vi "Save Config File.vi"(8 "error in (no error)":errorcluster, 10 "file path":path, 11 "DSF Configuration Reference in":T1) -> (0 "error out":errorcluster, 2 "file path out":path, 3 "DSF Configuration Reference out":T1)   [LabVIEW 2017, in "DSF Core.lvlib" / "Configuration Session.lvclass"]
uses:
  Configuration Session.lvclass
  Internal DSF Channel with ID.ctl
  Internal DSF Transfer with ID.ctl
  Typedefs/DSF Timing Info.ctl
  DSF Core.lvlib
  Internal DSF Group with ID.ctl
  Internal DSF Plugin with ID.ctl
  Typedefs/DSF Version Info.ctl
  Internal DSF Settings with ID.ctl
  Internal DSF Configuration.ctl
  Internal DSF Channel Info.ctl
  Internal DSF Transfer Info.ctl
  Internal DSF Group Info.ctl
  Internal DSF Plugin Info.ctl
  Internal DSF Settings Info.ctl
  DSF Config Data.ctl
  DSF Config Data Ref.ctl
  Typedefs/DSF Settings Info.ctl
  Typedefs/DSF Engine Plugin Thread Configuration.ctl
  Typedefs/DSF Engine Framework Configuration.ctl
  Typedefs/DSF Direction.ctl
  Typedefs/DSF Byte Order.ctl
  Typedefs/DSF Data Type.ctl
  Typedefs/DSF Engine Channel Configuration.ctl
  Typedefs/DSF Engine Transfer Configuration.ctl
  Typedefs/DSF Timeout Behavior.ctl
  Typedefs/DSF Engine Transfer Group Configuration.ctl
  Typedefs/DSF Engine Plugin Configuration.ctl
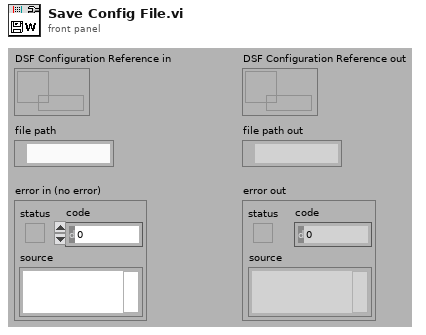
[diagram p1: front panel]
types:
  T1 = typedef "DSF Core.lvlib/Configuration Session.lvclass/DSF Config Data Ref.ctl" = refnum<data-value>
  T2 = enum16{"open", "replace", "create", "open or create", "replace or create", "replace or create with confirmation"}
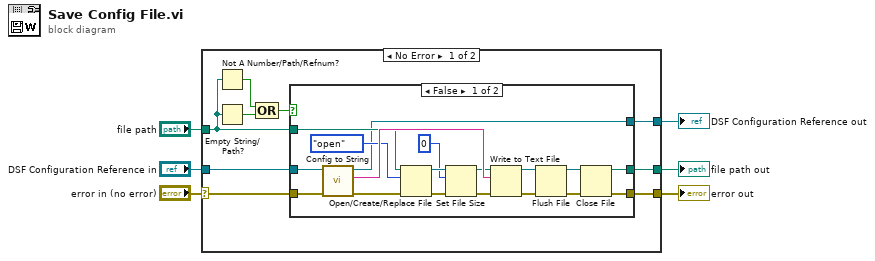
[diagram p0: block diagram]
diagram:
  n1 = case shown="No Error" "error in (no error)" {
    selector: "error in (no error)" -> [w8 w39]
    tunnel: [w15 w39] -> w5
    tunnel: [w14 w38] -> w3
    tunnel: "DSF Configuration Reference in" -> [w9 w38]
    tunnel: "file path" -> [w10 w37]
    tunnel: [w7 w37] -> w1
    frame No Error {
      n2 = Not A Number/Path/Refnum? ("Not A Number/Path/dsf refnum?")(number/path/refnum=w10) -> (NaN/Path/Refnum?=w13:bool)
      n3 = Empty String/Path?(string/path=w10) -> (empty?=w12:bool)
      n4 = Compound Arithmetic op=OR(w13, w12) -> (w11:bool)
      n5 = case shown="False" w11 {
        tunnel: [w32 w36] -> w15
        tunnel: w8 -> [w28 w36]
        tunnel: w10 -> [w29 w34]
        tunnel: w9 -> [w30 w35]
        tunnel: [w25 w35] -> w14
        tunnel: [w24 w34] -> w7
        frame False {
          n6 = call "Config to String.vi"("error in (no error)"=w28, "DSF Configuration Reference in"=w30) -> ("error out"=w27:errorcluster, "json string"=w31:string, "DSF Configuration Reference out"=w25:T1)  [unwired: 7 out]
          n7 = Open/Create/Replace File(file path (use dialog)=w29, error in=w27, operation (0:open)=T2."open") -> (refnum out=w21:refnum<file>, error out=w23:errorcluster)  [unwired: 4 out]
          n8 = Set File Size(4:w23, 6:i64 0 ("size (in bytes)"), 7:w21) -> (0:w22:errorcluster, 3:w20:refnum<file>)
          n9 = Write to Text File(file (use dialog)=w20, text=w31, error in=w22) -> (refnum out=w17:refnum<file>, error out=w33:errorcluster)  [unwired: 2 out]
          n10 = Flush File(refnum=w17, error in=w33) -> (refnum out=w16:refnum<file>, error out=w18:errorcluster)
          n11 = Close File(refnum=w16, error in=w18) -> (path=w24:path, error out=w32:errorcluster)
        }
        frame True {
        }
      }
    }
    frame Error {
    }
  }
  "error out" <- w5
  "DSF Configuration Reference out" <- w3
  "file path out" <- w1
